vi "CRYRename Dialog.vi"(6 "sAction":string, 9 "Type":enum16{"Curves", "Values", "Results", "WFM"}(ring), 10 "Name In":string[](array[string])) -> (0 "bReturn":bool, 1 "Org Name":string[](array[string]), 2 "Index":i32, 3 "New Name":string[](array[string]))   [LabVIEW 2013]
panel:
  in  "Cancel":bool
  in  "OK":bool
  in  "Name":string
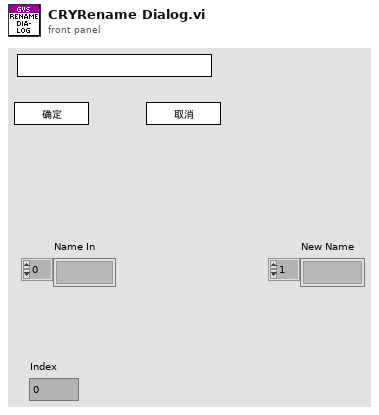
[diagram p1: front panel]
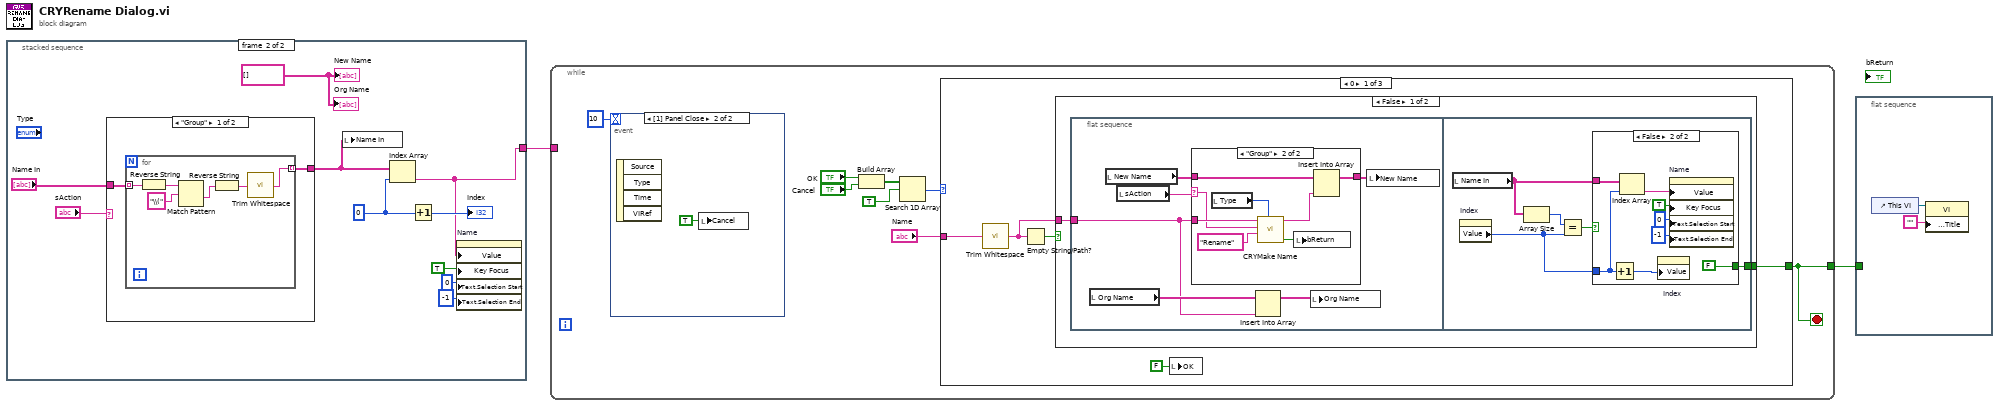
[diagram p0: block diagram]
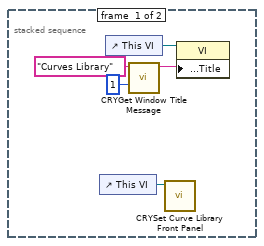
[diagram p2: hidden frame]
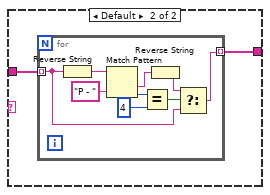
[diagram p3: hidden frame]
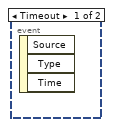
[diagram p4: hidden frame]
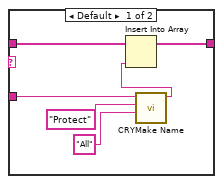
[diagram p5: hidden frame]
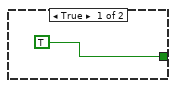
[diagram p6: hidden frame]
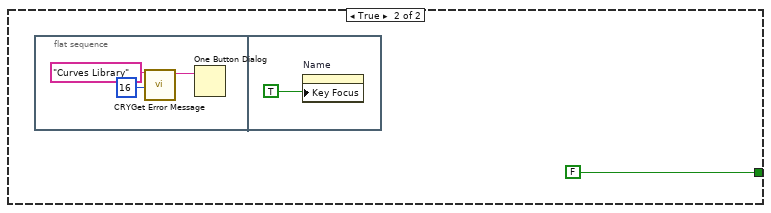
[diagram p7: hidden frame]
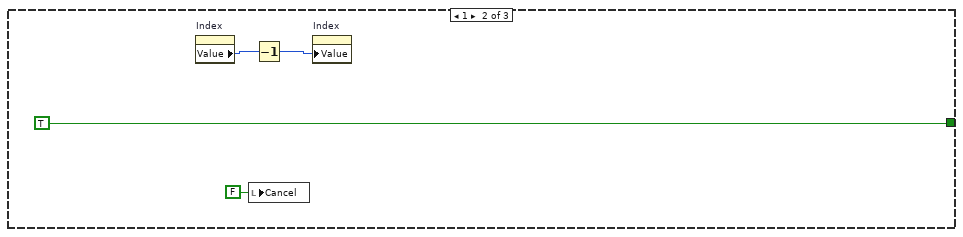
[diagram p8: hidden frame]
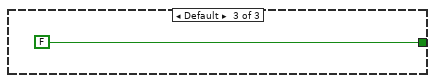
[diagram p9: hidden frame]
diagram:
  n1 = stacked-sequence {
    tunnel: [_ w14] -> w2
    frame #0 {
      n2 = control-ref of="This VI"() -> (w4:refnum<vi>)
      n3 = control-ref of="This VI"() -> (w5:refnum<vi>)
      n4 = call "CRYGet Window Title Message.vi"("No"=1 ("Error No"), "Kind"="Curves Library") -> ("Multibyte String"=w3:string)  [unwired: 4 in, 5 out]
      n5 = call "CRYSet Curve Library Front Panel.vi"("Vi Ref In"=w4) -> ()  [unwired: 10 in, 1 out]
      n6 = property class="VI"(reference=w5, "Front Panel.Title"=w3) -> ()  [unwired: 1 in, 2 out]
    }
    frame #1 {
      w17 = 0 ("Index")
      w8 = string[] [] ("Name In")
      n7 = case shown="\"Group\"" "sAction" {
        tunnel: "Name In" -> [w19 w27]
        tunnel: [w18 w26] -> w13
        frame "Group" {
          n8 = for {
            tunnel: [w20] -> w18 mode=indexing
            tunnel: w19 -> [w22] mode=indexing
            n9 = Reverse String(1:w22) -> (0:w25:string)
            n10 = Match Pattern(string=w25, regular expression="\\(" ("search string/char (-)")) -> (after substring=w23:string)  [unwired: 1 in, 3 out]
            n11 = Reverse String(1:w23) -> (0:w21:string)
            n12 = call <vilib>:"Trim Whitespace.vi"("string"=w21) -> ("trimmed string"=w20:string)  [unwired: 1 in]
          }
        }
        frame Default {
          n13 = for {
            tunnel: [w31] -> w26 mode=indexing
            tunnel: w27 -> [w28] mode=indexing
            n14 = Reverse String(1:w28) -> (0:w36:string)
            n15 = Match Pattern(string=w36, regular expression="P - " ("search string/char (-)")) -> (after substring=w30:string, offset past match=w33:i32)  [unwired: 1 in, 2 out]
            n16 = Equal?(x=w33, y=4) -> (x = y?=w34:bool)
            n17 = Reverse String(1:w30) -> (0:w29:string)
            n18 = Select(t=w29, s=w34, f=w28) -> (s? t:f=w31:string)
          }
        }
      }
      n19 = local write "Name In"(w13) -> ()
      n20 = Index Array(array=w13, index=w17) -> (element=w14:string)
      n21 = Increment(x=w17) -> (x+1=→"Index":i32)
      n22 = property on="Name" class="Str"("Value"=w14, "Key Focus"=TRUE, "Text.Selection Start"=u32 0 ("Text.Selection:Start"), "Text.Selection End"=-1) -> ()  [unwired: 2 in, 2 out]
      "New Name" <- w8
      "Org Name" <- w8
    }
  }
  n23 = while {
    tunnel: w2 -> [_]
    tunnel: [w39] -> w1
    stop <- w39 stop-if-true
    n24 = event shown="[1] Panel Close" {
      selector: _ -> [_ _]
      dyn-events: _ -> [_ _]
      timeout: 10 -> [_ _]
      event Timeout {
        n25 = event-data() -> ()  [unwired: 1 in, 3 out]
      }
      event Panel Close {
        n26 = event-data() -> ()  [unwired: 1 in, 4 out]
        n27 = local write "Cancel"(TRUE ("Cancel")) -> ()
      }
    }
    n28 = Build Array("OK", "Cancel") -> (w42:bool[])
    n29 = Search 1D Array(1D array=w42, element=TRUE) -> (index of element=w40:i32)  [unwired: 1 out]
    n30 = case shown="0" w40 {
      tunnel: [w50 TRUE FALSE] -> w39
      tunnel: "Name" -> [w48 _ _]
      frame 0 {
        n31 = call <vilib>:"Trim Whitespace.vi"("string"=w48) -> ("trimmed string"=w46:string)  [unwired: 1 in]
        n32 = Empty String/Path?(string/path=w46) -> (empty?=w47:bool)
        n33 = case shown="False" w47 {
          tunnel: [w52 FALSE] -> w50
          tunnel: w46 -> [w51 _]
          frame False {
            n34 = flat-sequence {
              tunnel: w51 -> [w53]
              tunnel: [w75] -> w52
              frame #0 {
                n35 = local read "Org Name"() -> (w55:string[])
                n36 = local read "New Name"() -> (w57:string[])
                n37 = local read "sAction"() -> (w56:string)
                n38 = case shown="\"Group\"" w56 {
                  selector: w56 -> [_ w68]
                  tunnel: [w64 w72] -> w58
                  tunnel: w57 -> [w63 w71]
                  tunnel: w53 -> [w59 w69]
                  frame Default {
                    n39 = call "CRYMake Name.vi"("sOption"="All", "sAction"="Protect" ("sOption"), "Name In"=w59) -> ("Name Out"=w62:string)  [unwired: 7 in, 1 out]
                    n40 = Insert Into Array(array=w63, new element=w62) -> (w64:string[])  [unwired: 1 in]
                  }
                  frame "Group" {
                    n41 = local read "Type"() -> (w65:enum16{"Curves", "Values", "Results", "WFM"})
                    n42 = call "CRYMake Name.vi"("Type"=w65, "sOption"="Rename", "sAction"=w68, "Name In"=w69) -> ("Exist?"=w66:bool, "Name Out"=w70:string)  [unwired: 6 in]
                    n43 = local write "bReturn"(w66) -> ()
                    n44 = Insert Into Array(array=w71, new element=w70) -> (w72:string[])  [unwired: 1 in]
                  }
                }
                n45 = Insert Into Array(array=w55, new element=w53) -> (w54:string[])  [unwired: 1 in]
                n46 = local write "Org Name"(w54) -> ()
                n47 = local write "New Name"(w58) -> ()
              }
              frame #1 {
                n48 = local read "Name In"() -> (w74:string[])
                n49 = property on="Index" class="DigNum (strict)"() -> ("Value"=w73:i32)  [unwired: 2 in, 2 out]
                n50 = Array Size(array=w74) -> (size(s)=w77:i32)
                n51 = Equal?(x=w77, y=w73) -> (x = y?=w76:bool)
                n52 = case shown="False" w76 {
                  tunnel: [TRUE FALSE] -> w75
                  tunnel: w73 -> [_ w84]
                  tunnel: w74 -> [_ w86]
                  frame True {
                  }
                  frame False {
                    n53 = Increment(x=w84) -> (x+1=w83:i32)
                    n54 = Index Array(array=w86, index=w84) -> (element=w79:string)
                    n55 = property on="Index" class="DigNum (strict)"("Value"=w83) -> ()  [unwired: 2 in, 2 out]
                    n56 = property on="Name" class="Str"("Value"=w79, "Key Focus"=TRUE, "Text.Selection Start"=u32 0 ("Text.Selection:Start"), "Text.Selection End"=-1) -> ()  [unwired: 2 in, 2 out]
                  }
                }
              }
            }
          }
          frame True {
            n57 = flat-sequence {
              frame #0 {
                n58 = call "CRYGet Error Message.vi"("Error No"=16 ("No"), "Kind"="Curves Library") -> ("Message"=w90:string)  [unwired: 4 in, 5 out]
                n59 = One Button Dialog(message=w90) -> ()  [unwired: 2 out]
              }
              frame #1 {
                n60 = property on="Name" class="Str"("Key Focus"=TRUE) -> ()  [unwired: 2 in, 2 out]
              }
            }
          }
        }
        n61 = local write "OK"(FALSE ("OK")) -> ()
      }
      frame 1 {
        n62 = property on="Index" class="DigNum (strict)"() -> ("Value"=w94:i32)  [unwired: 2 in, 2 out]
        n63 = local write "Cancel"(FALSE ("Cancel")) -> ()
        n64 = Decrement(x=w94) -> (x-1=w93:i32)
        n65 = property on="Index" class="DigNum (strict)"("Value"=w93) -> ()  [unwired: 2 in, 2 out]
      }
      frame Default {
      }
    }
  }
  n66 = flat-sequence {
    tunnel: w1 -> [_]
    frame #0 {
      n67 = control-ref of="This VI"() -> (w98:refnum<vi>)
      n68 = property class="VI"(reference=w98, "Front Panel.Title"="") -> ()  [unwired: 1 in, 2 out]
    }
  }
